vi "Actor Core.vi"(8 "error in":errorcluster caption="错误输入", 11 "下位机":refnum<class "下位机模拟.lvclass"> caption="操作者输入") -> (0 "error out":errorcluster caption="错误输出", 3 "Actor out":refnum<class "Actor.lvclass"> caption="操作者输出")   [LabVIEW 2015, in "下位机模拟.lvlib" / "下位机模拟.lvclass"]
doc: "(<B>Filename</B>: Actor Framework.lvlib:Actor.lvclass:Actor Core.vi)\n\nReceives messages to the actor, reacts to them, and initiates any error handling that may shut the actor down.\n\nDescendant classes may override this VI to append parallel tasks for the actor to complete while it handles messages. Overrides use the Call Parent Method node."
uses:
  <vilib>/ActorFramework/Actor/Actor.lvclass
panel:
  in  "发送数据列表":i32(listbox)
  out "接收数据列表":i32(listbox)
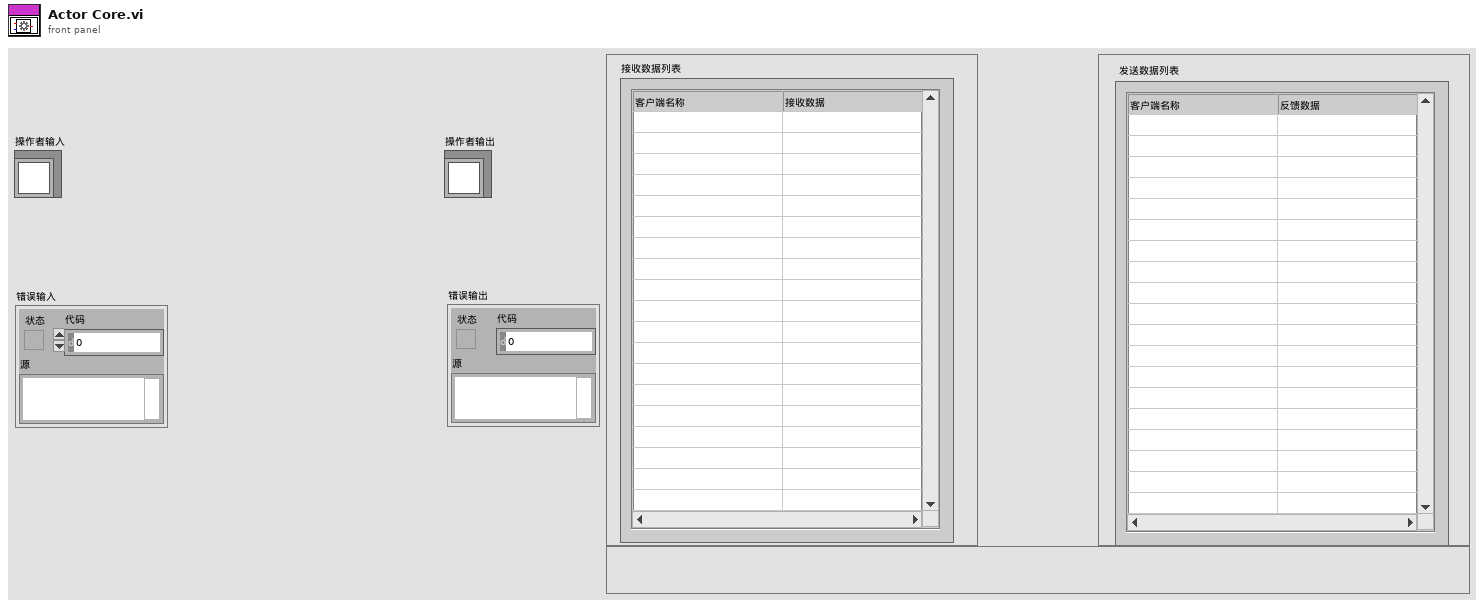
[diagram p1: front panel]
types:
  T1 = cluster{"接收数据列表":string[][], "发送数据列表":string[][]}
  T2 = typedef "LVRowAndColumnUnsignedTypeDef.ctl" = cluster{"Row":u32, "Column":u32}
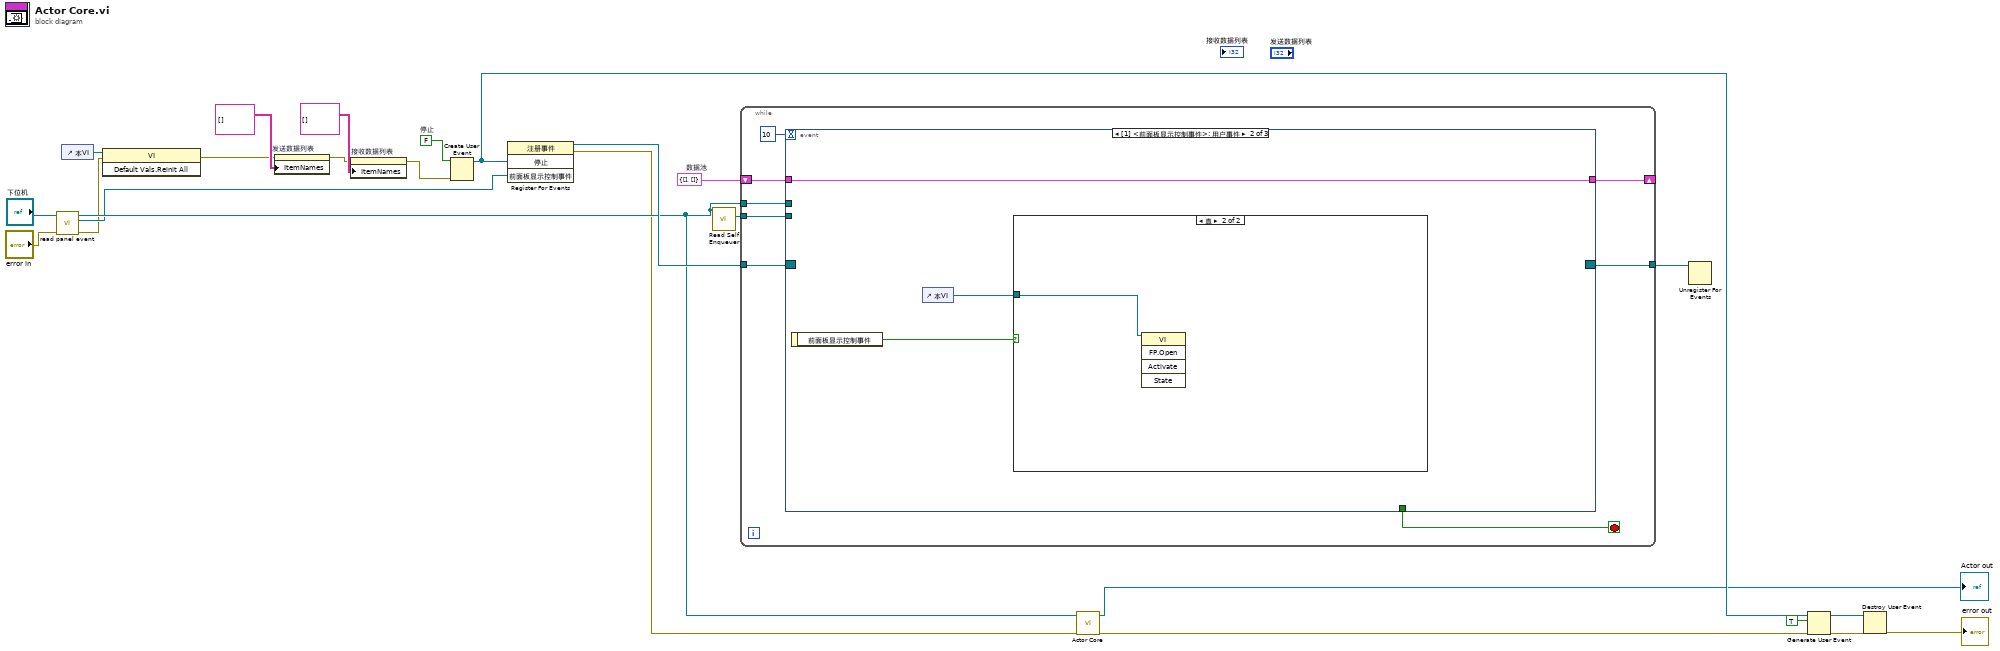
[diagram p0: block diagram]
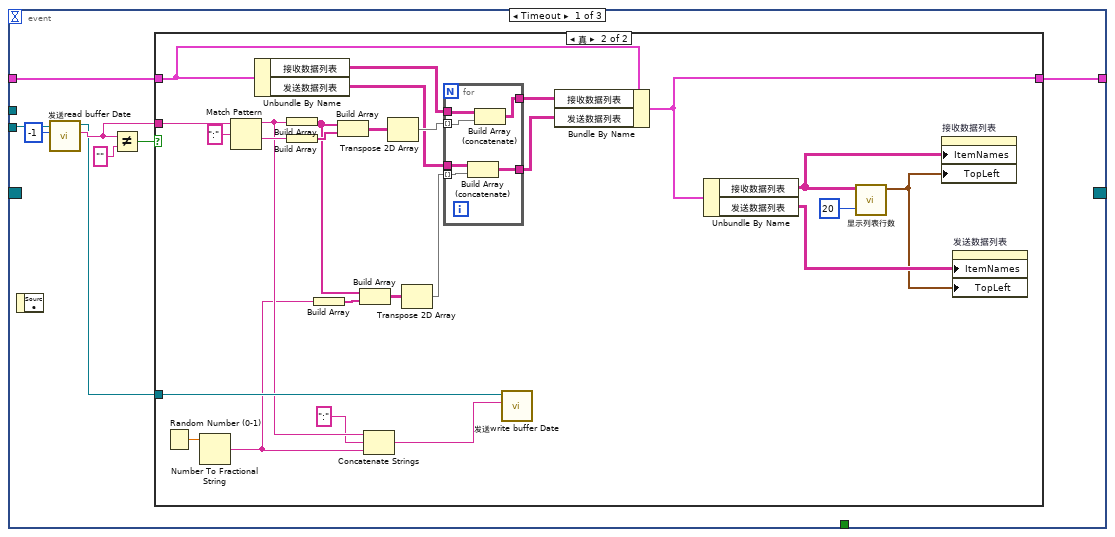
[diagram p2: hidden frame]
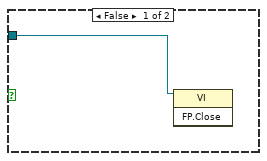
[diagram p4: hidden frame]
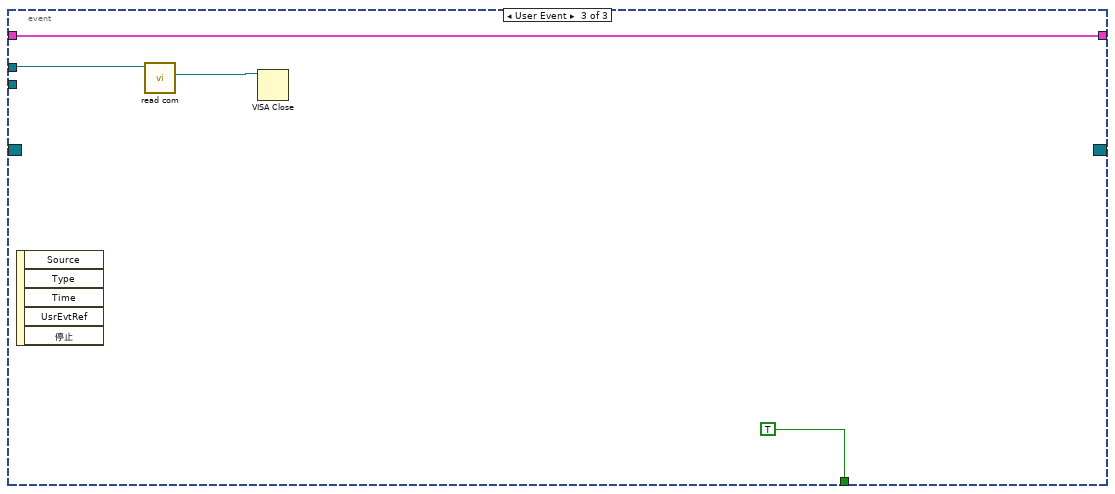
[diagram p5: hidden frame]
diagram:
  w22 = FALSE  # 停止
  w23 = T1 {"接收数据列表"=[], "发送数据列表"=[]}  # 数据池
  n1 = call "read panel event.vi"("error in (no error)"="error in", "前面板控制 输入"="下位机") -> ("error out"=w10:errorcluster, "前面板显示控制事件"=w13:refnum<user-event>, "前面板控制 输出"=w14:refnum<class "下位机模拟.lvclass">)  [unwired: 7 in]
  n2 = control-ref of="本VI"() -> (w11:refnum<vi>)
  n3 = invoke class="VI" method="Default Vals.Reinit All"(reference=w11, error in=w10) -> (error out=w5:errorcluster)  [unwired: 1 in, 2 out]
  n4 = property on="发送数据列表" class="MCListbox (严格)"(error in=w5, "ItemNames"=string[][] [] ("项名")) -> (error out=w6:errorcluster)  [unwired: 1 in, 1 out]
  n5 = property on="接收数据列表" class="MCListbox (严格)"(error in=w6, "ItemNames"=string[][] [] ("项名")) -> (error out=w4:errorcluster)  [unwired: 1 in, 1 out]
  n6 = Create User Event(user event datatype=w22, error in=w4) -> (user event=w19:refnum<user-event>)  [unwired: 1 out]
  n7 = register-events(w19, w13) -> (reference out=w21:refnum<event-registration>, error out=w12:errorcluster)  [unwired: 2 in]
  n8 = call <vilib>:"Read Self Enqueuer.vi"("Actor"=w14) -> ("Self Enqueuer"=w24:refnum<class "Message Enqueuer.lvclass">)  [unwired: 10 in]
  n9 = while {
    tunnel: w24 -> [w32]
    shift-right: [w30] -> _
    shift-left: w23 -> [w31]
    tunnel: w21 -> [w28]
    tunnel: [w27] -> w20
    tunnel: w14 -> [w25]
    stop <- w29 stop-if-true
    n10 = event shown="[1] <前面板显示控制事件>: 用户事件" {
      selector: w28 -> [_ _ _]
      dyn-events: [_ _ _] -> w27
      timeout: 10 -> [_ _ _]
      tunnel: w32 -> [w36 _ _]
      tunnel: w31 -> [w38 w74 w79]
      tunnel: [w37 w74 w79] -> w30
      tunnel: [_ _ TRUE] -> w29
      tunnel: w25 -> [_ _ w80]
      event Timeout {
        n11 = event-data() -> ()  [unwired: 1 in, 1 out]
        n12 = call "发送read buffer Date.vi"("timeout in ms (-1)"=-1, "Message Enqueuer"=w36) -> ("read buffer date"=w34:string, "Message Enqueuer out"=w33:refnum<class "Message Enqueuer.lvclass">)  [unwired: 7 in, 1 out]
        n13 = Not Equal?(x=w34, y="") -> (x != y?=w39:bool)
        n14 = case shown="真" w39 {
          tunnel: w38 -> [w41 w61]
          tunnel: [w41 w59] -> w37
          tunnel: w34 -> [_ w50]
          tunnel: w33 -> [_ w49]
          frame False {
          }
          frame True {
            n15 = Random Number (0-1)() -> (number: 0 to 1=w56:dbl)
            n16 = Number To Fractional String(number=w56) -> (F-format string=w46:string)  [unwired: 3 in]
            n17 = Match Pattern(string=w50, regular expression=":" ("正则表达式")) -> (before substring=w48:string, after substring=w66:string)  [unwired: 1 in, 2 out]
            n18 = Unbundle By Name(w61) -> ("接收数据列表"=w62:string[][], "发送数据列表"=w44:string[][])
            n19 = Build Array(w48) -> (w55:string[])
            n20 = Build Array(w66) -> (w65:string[])
            n21 = Build Array(w46) -> (w54:string[])
            n22 = Build Array(w55, w65) -> (w64:string[][])
            n23 = Build Array(w55, w54) -> (w53:string[][])
            n24 = Concatenate Strings(w48, ":" ("正则表达式"), w46) -> (w45:string)
            n25 = Transpose 2D Array(2D array=w64) -> (transposed array=w63:string[][])
            n26 = Transpose 2D Array(2D array=w53) -> (transposed array=w42:string[][])
            n27 = for {
              tunnel: w63 -> [w73] mode=indexing
              tunnel: [w72] -> w60
              tunnel: w62 -> [w71]
              tunnel: w44 -> [w70]
              tunnel: [w69] -> w43
              tunnel: w42 -> [w68] mode=indexing
              n28 = Build Array (concatenate)(w70, w68) -> (w69:string[][])
              n29 = Build Array (concatenate)(w71, w73) -> (w72:string[][])
            }
            n30 = call "发送write buffer Date.vi"("写入缓冲区"=w45, "Message Enqueuer"=w49) -> ()  [unwired: 8 in, 2 out]
            n31 = Bundle By Name(cluster=w61, "接收数据列表"=w60, "发送数据列表"=w43) -> (w59:T1)
            n32 = Unbundle By Name(w59) -> ("接收数据列表"=w58:string[][], "发送数据列表"=w52:string[][])
            n33 = call "显示列表行数.vi"("显示行数"=20, "接收数据列表"=w58) -> ("输出簇"=w51:T2)  [unwired: 9 in]
            n34 = property on="接收数据列表" class="MCListbox (严格)"("ItemNames"=w58, "TopLeft"=w51) -> ()  [unwired: 2 in, 2 out]
            n35 = property on="发送数据列表" class="MCListbox (严格)"("ItemNames"=w52, "TopLeft"=w51) -> ()  [unwired: 2 in, 2 out]
          }
        }
      }
      event User Event {
        n36 = event-data() -> ("前面板显示控制事件"=w76:bool)  [unwired: 1 in]
        n37 = control-ref of="本VI"() -> (w75:refnum<vi>)
        n38 = case shown="真" w76 {
          tunnel: w75 -> [w77 w78]
          frame False {
            n39 = invoke class="VI" method="FP.Close"(reference=w77) -> ()  [unwired: 2 in, 3 out]
          }
          frame True {
            n40 = invoke class="VI" method="FP.Open"(reference=w78) -> ()  [unwired: 4 in, 5 out]
          }
        }
      }
      event User Event {
        n41 = event-data() -> ()  [unwired: 1 in, 5 out]
        n42 = call "read com.vi"("串口参数管理 输入"=w80) -> ("COM"=w81:refnum<visa-resource-name>)  [unwired: 8 in, 2 out]
        n43 = VISA Close(VISA resource name=w81) -> ()  [unwired: 1 in, 1 out]
      }
    }
  }
  n44 = call-parent "Actor Core.vi"("error in"=w12, "Actor in"=w14) -> ("error out"=w18:errorcluster, "Actor out"=→"Actor out":refnum<class "Actor.lvclass">)  [unwired: 8 in]
  n45 = Unregister For Events(event registration refnum=w20) -> ()  [unwired: 1 in, 1 out]
  n46 = Generate User Event(user event=w19, event data cluster=TRUE, error in=w18) -> (user event out=w2:refnum<user-event>, error out=w1:errorcluster)  [unwired: 1 in]
  n47 = Destroy User Event(user event=w2, error in=w1) -> (error out=→"error out":errorcluster)
